vi "ConfigUtilities - Tx or Rx.vi"(8 "error in (no error)":errorcluster, 11 "Item Ref in":T1 format="%.0x") -> (0 "error out":errorcluster, 2 "Tx?":bool, 3 "Item Ref out":T1 format="%.0x")   [LabVIEW 2016, in "UDP-Custom-Device System Explorer.lvlib"]
uses:
  UDP-Custom-Device System Explorer.lvlib
  <vilib>/NI Veristand/Custom Device API/Custom Device Item Ref.ctl
  <vilib>/NI VeriStand/Custom Device API/Custom Device API.lvlib
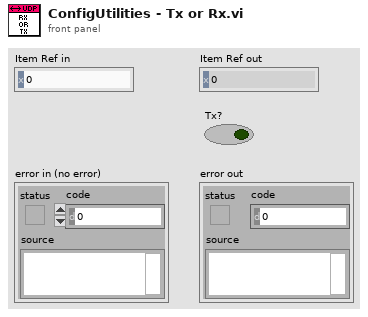
[diagram p1: front panel]
types:
  T1 = typedef "Custom Device API.lvlib/Custom Device Item Ref.ctl" = u64
  T2 = typedef "Custom Device API.lvlib/Custom Device Item Info.ctl" = cluster{"Name":string, "Is Channel":bool, "GUID":string, "Is Waveform":bool}
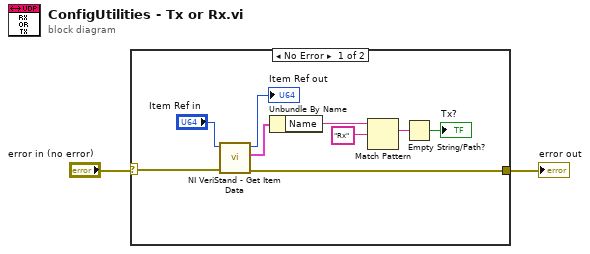
[diagram p0: block diagram]
diagram:
  n1 = case shown="No Error" "error in (no error)" {
    selector: "error in (no error)" -> [w5 w12]
    tunnel: [w7 w12] -> w2
    frame No Error {
      n2 = call <vilib>:"NI VeriStand - Get Item Data.vi"("error in (no error)"=w5, "Item Ref in"="Item Ref in") -> ("error out"=w7:errorcluster, "Item Info"=w9:T2, "Item Ref out"=→"Item Ref out":T1)  [unwired: 6 in, 1 out]
      n3 = Unbundle By Name(w9) -> ("Name"=w4:string)
      n4 = Match Pattern(string=w4, regular expression="Rx") -> (match substring=w3:string)  [unwired: 1 in, 3 out]
      n5 = Empty String/Path?(string/path=w3) -> (empty?=→"Tx?":bool)
    }
    frame Error {
    }
  }
  "error out" <- w2
